vi "ContRunMainDEBUG.vi"(8 "error in (no error)":errorcluster, 9 "step num":dbl, 10 "runs slider ref":refnum<vi>, 11 "Main pulse seq":T2) -> (0 "error out":errorcluster, 3 "readout":T1, 5 "Stop":bool)   [LabVIEW 2019]
uses:
  PulseControl.ctl
  Compiler/Params.ctl
  controls/GlobalExp.vi
  <vilib>/gmath/statdist.llb/Normal PDF.vi
  <vilib>/gmath/statdist.llb/Normal Random.vi
  Global.lvlib
  <vilib>/gmath/NI_Gmath.lvlib
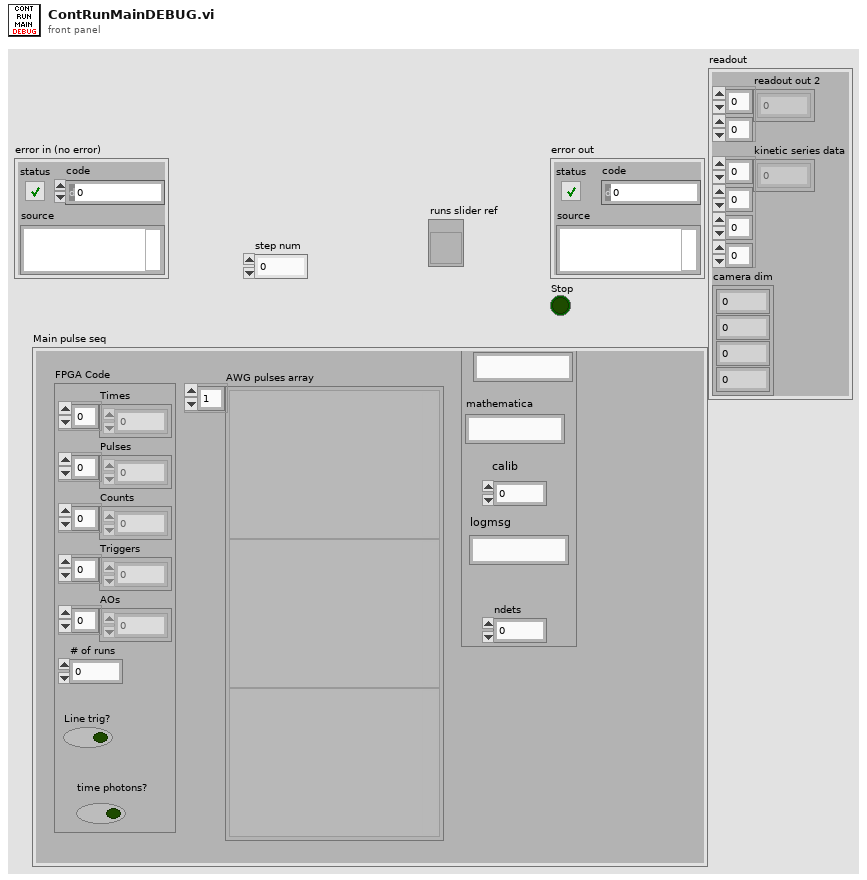
[diagram p1: front panel]
types:
  T1 = cluster{"readout out 2":dbl[][], "kinetic series data":i32[][][][], "camera dim":cluster{i32, i32, i32, i32}}
  T2 = typedef "PulseControl.ctl" = cluster{"FPGA Code":cluster{"Times":u32[], "Pulses":u64[], "Counts":u8[], "Triggers":u8[], "AOs":u8[], "# of runs":i32, "Line trig?":bool, "time photons?":bool}, "AWG pulses array":variant[], "Params":T3}
  T3 = typedef "Params.ctl" = cluster{"steps":i16, "runs":i16, "comment":string, "mathematica":string, "calib":i8, "logmsg":string, "ndets":i16}
  T4 = cluster{"runs":i32, "readouts":i32, "width":i32, "height":i32}
  T5 = cluster{"readout out 2":i32[][], "kinetic series data":i32[][][][], "camera dim":cluster{i32, i32, i32, i32}}
  T6 = enum16{"Innit", "Stop", "Idle", "MainRunning", "AuxRunning"}
  T7 = typedef "MasterExpControl.ctl" = cluster{"Main Steps":dbl, "Main Runs":dbl, "ExpStatus":enum16{"Innit", "Stop", "Idle", "MainRunning", "AuxRunning"}, "Main Current Step":dbl, "ExpNum":dbl, "NewData":bool, "date":string, "command":string, "Stop":bool, "Pause":bool, "Mathematica":string, "Main/Meta":bool, "UpdateMath":bool, "Camera":bool, "MetaExpOver":bool, "NextMetaExp":bool}
  T8 = enum16{"twobright", "rightbright", "leftbright", "dark"}
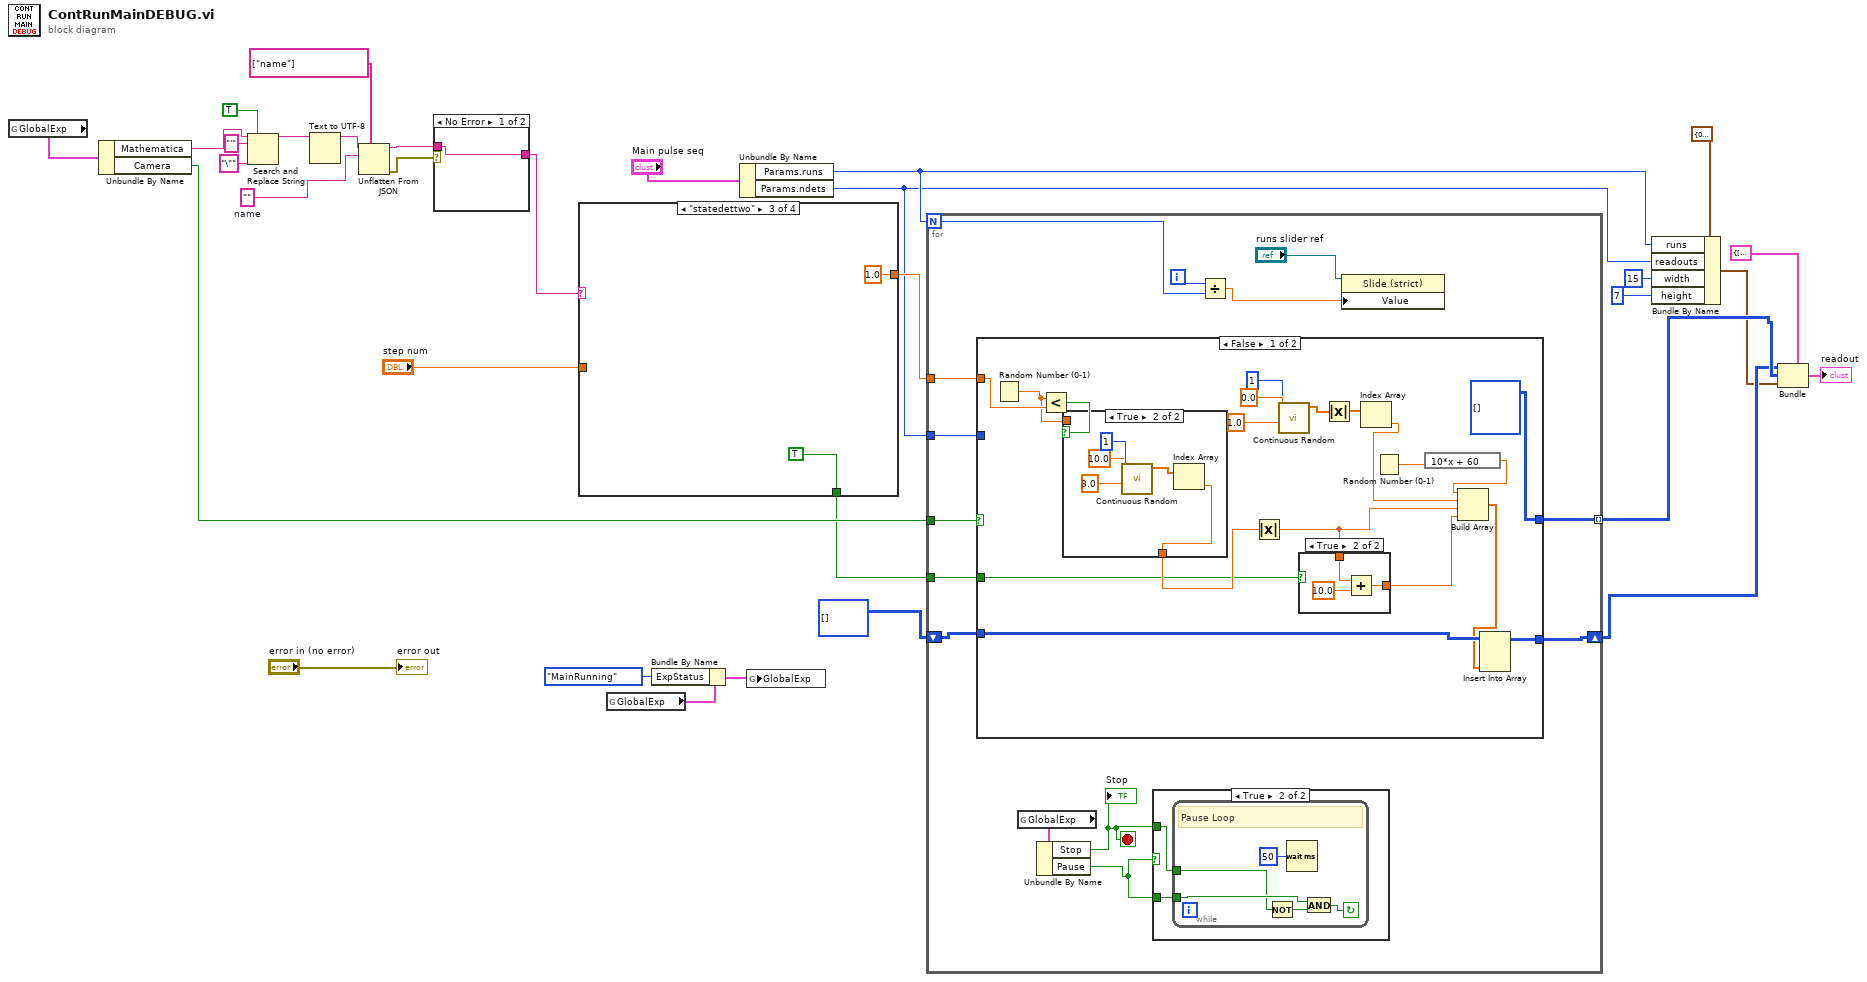
[diagram p0: block diagram]
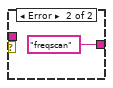
[diagram p2: hidden frame]
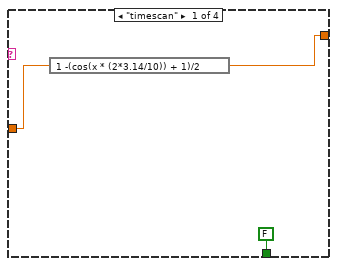
[diagram p3: hidden frame]
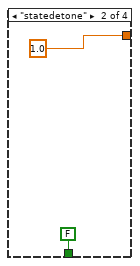
[diagram p4: hidden frame]
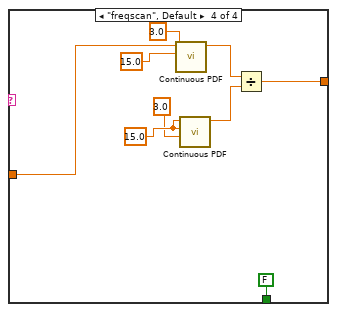
[diagram p5: hidden frame]
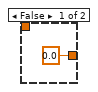
[diagram p6: hidden frame]
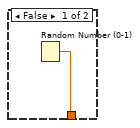
[diagram p7: hidden frame]
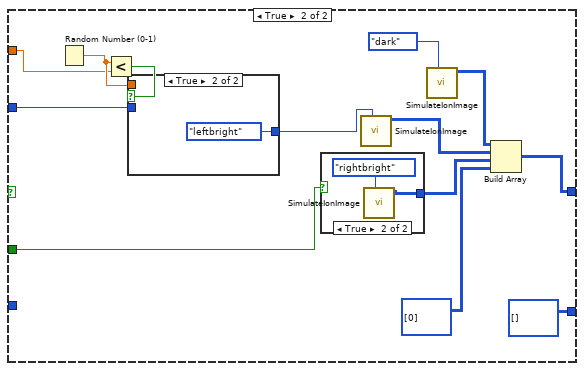
[diagram p8: hidden frame]
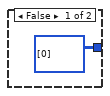
[diagram p9: hidden frame]
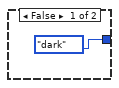
[diagram p10: hidden frame]
diagram:
  w18 = ""  # name
  n1 = global read "GlobalExp.vi" "GlobalExp"() -> (w25:T7)
  n2 = Unbundle By Name(w25) -> ("Mathematica"=w24:string, "Camera"=w11:bool)
  n3 = Search and Replace String(replace all?=TRUE ("replace all? (F)"), input string=w24, search string="'", replace string="\"" ("replace string (\"\")")) -> (result string=w19:string)  [unwired: 4 in, 3 out]
  n4 = Text to UTF-8(11:w19) -> (3:w23:string)  [unwired: 2 in, 1 out]
  n5 = Unflatten From JSON(path=string[] ["name"], JSON string=w23, type and defaults=w18) -> (value=w15:string, error out=w16:errorcluster)  [unwired: 4 in]
  n6 = case shown="No Error" w16 {
    tunnel: [w33 "freqscan" ("name")] -> w14
    tunnel: w15 -> [w33 _]
    frame No Error {
    }
    frame Error {
    }
  }
  n7 = case shown="\"statedettwo\"" w14 {
    tunnel: "step num" -> [w36 _ _ w44]
    tunnel: [w37 1.0 ("step num") 1.0 ("step num") w43] -> w26
    tunnel: [FALSE FALSE TRUE FALSE] -> w1
    frame "timescan" {
      n8 = expression code="1 -(cos(x * (2*3.14/10)) + 1)/2"(w36) -> (w37:dbl)
    }
    frame "statedetone" {
    }
    frame "statedettwo" {
    }
    frame "freqscan", Default {
      w48 = 15.0 ("mean")
      n9 = call-poly <vilib>:"Continuous PDF.vi"("std"=3.0, "mean"=15.0, "x"=w44) -> ("pdf(x)"=w49:dbl)  [unwired: 7 in, 1 out]
      n10 = call-poly <vilib>:"Continuous PDF.vi"("std"=3.0, "mean"=w48, "x"=w48) -> ("pdf(x)"=w50:dbl)  [unwired: 7 in, 1 out]
      n11 = Divide(x=w49, y=w50) -> (x/y=w43:dbl)
    }
  }
  n12 = global read "GlobalExp.vi" "GlobalExp"() -> (w31:T7)
  n13 = Bundle By Name(cluster=w31, "ExpStatus"=T6."MainRunning") -> (w30:T7)
  n14 = Unbundle By Name("Main pulse seq") -> ("Params.runs"=w6:i16, "Params.ndets"=w5:i16)
  n15 = global write "GlobalExp.vi" "GlobalExp"(w30) -> ()
  n16 = for {
    N: w6 -> [w63]
    tunnel: w26 -> [w57]
    tunnel: w11 -> [w56]
    tunnel: w5 -> [w55]
    tunnel: [w54] -> w10 mode=indexing
    shift-right: [w52] -> w8
    shift-left: i32[][] [] -> [w53]
    tunnel: w1 -> [w51]
    i -> [w64]
    stop <- w59 stop-if-true
    n17 = case shown="False" w56 {
      tunnel: w53 -> [w81 _]
      tunnel: [w79 i32[][] []] -> w52
      tunnel: w57 -> [w78 w104]
      tunnel: w55 -> [_ w103]
      tunnel: [i32[][][] [] w97] -> w54
      tunnel: w51 -> [w65 w94]
      frame False {
        n18 = Random Number (0-1)() -> (number: 0 to 1=w76:dbl)
        n19 = Less?(x=w76, y=w78) -> (x < y?=w77:bool)
        n20 = case shown="True" w77 {
          tunnel: [w88 w89] -> w69
          tunnel: w76 -> [_ _]
          frame False {
            n21 = Random Number (0-1)() -> (number: 0 to 1=w88:dbl)
          }
          frame True {
            n22 = call-poly <vilib>:"Continuous Random.vi"("std"=3.0, "mean"=10.0, "samples"=1) -> ("normal random data"=w90:dbl[])  [unwired: 7 in, 1 out]
            n23 = Index Array(array=w90) -> (element=w89:dbl)  [unwired: 1 in]
          }
        }
        n24 = Absolute Value(x=w69) -> (abs(x)=w66:dbl)
        n25 = call-poly <vilib>:"Continuous Random.vi"("std"=1.0, "mean"=0.0, "samples"=1) -> ("normal random data"=w73:dbl[])  [unwired: 7 in, 1 out]
        n26 = case shown="True" w65 {
          tunnel: [0.0 w87] -> w67
          tunnel: w66 -> [_ w85]
          frame False {
          }
          frame True {
            n27 = Add(x=w85, y=10.0) -> (x+y=w87:dbl)
          }
        }
        n28 = Absolute Value(x=w73) -> (abs(x)=w71:dbl[])
        n29 = Index Array(array=w71) -> (element=w70:dbl)  [unwired: 1 in]
        n30 = Random Number (0-1)() -> (number: 0 to 1=w83:dbl)
        n31 = expression code="10*x + 60"(w83) -> (w82:dbl)
        n32 = Build Array(w82, w70, w66, w67) -> (w80:dbl[])
        n33 = Insert Into Array(array=w81, new element=w80) -> (w79:i32[][])  [unwired: 2 in]
      }
      frame True {
        n34 = Random Number (0-1)() -> (number: 0 to 1=w105:dbl)
        n35 = Less?(x=w105, y=w104) -> (x < y?=w106:bool)
        n36 = case shown="True" w106 {
          tunnel: w105 -> [_ _]
          tunnel: w103 -> [_ _]
          tunnel: [T8."dark" ("Enum") T8."leftbright" ("Enum")] -> w101
          frame False {
          }
          frame True {
          }
        }
        n37 = case shown="True" w94 {
          tunnel: [i32[][] [[0]] ("Intensity Graph") w109] -> w95
          frame False {
          }
          frame True {
            n38 = call "SimulateIonImage.vi"("Enum"=T8."rightbright") -> ("Intensity Graph"=w109:i32[][])  [unwired: 10 in]
          }
        }
        n39 = call "SimulateIonImage.vi"("Enum"=w101) -> ("Intensity Graph"=w100:i32[][])  [unwired: 10 in]
        n40 = call "SimulateIonImage.vi"("Enum"=T8."dark") -> ("Intensity Graph"=w99:i32[][])  [unwired: 10 in]
        n41 = Build Array(w99, w100, w95, i32[][] [[0]] ("element")) -> (w97:i32[][][])
      }
    }
    n42 = global read "GlobalExp.vi" "GlobalExp"() -> (w60:T7)
    n43 = Unbundle By Name(w60) -> ("Stop"=w59:bool, "Pause"=w58:bool)
    "Stop" <- w59
    n44 = case shown="True" w58 {
      tunnel: w58 -> [_ w113]
      tunnel: w59 -> [_ w112]
      frame False {
      }
      frame True {
        n45 = while {
          tunnel: w113 -> [w116]
          tunnel: w112 -> [w115]
          stop <- w114 continue-if-true
          # "Pause Loop"
          n46 = Not(x=w115) -> (.not. x?=w117:bool)
          n47 = Wait (ms)(milliseconds to wait=u32 50) -> ()  [unwired: 1 out]
          n48 = And(x=w116, y=w117) -> (x .and. y?=w114:bool)
        }
      }
    }
    n49 = Divide(x=w64, y=w63) -> (x/y=w61:dbl)
    n50 = property class="Slide (strict)"(reference="runs slider ref", "Value"=w61) -> ()  [unwired: 1 in, 2 out]
  }
  n51 = Bundle By Name(cluster=T4 {"runs"=0, "readouts"=0, "width"=0, "height"=0} ("camera dim"), "runs"=w6, "readouts"=w5, "width"=15, "height"=7) -> (w2:T4)
  n52 = Bundle(cluster=T5 {"readout out 2"=[], "kinetic series data"=[], "camera dim"={0, 0, 0, 0}} ("readout 3"), "readout out 2"=w8, "kinetic series data"=w10, "camera dim"=w2) -> (→"readout":T5)
  "error out" <- "error in (no error)"
